vi "HowManyHours.vi"(1 "Error In":errorcluster, 2 "Money":dbl=30.8 format="%#_13g") -> (0 "Info":string)   [LabVIEW 2023]
panel:
  in  "zakończ":bool
  out "Error Out":errorcluster
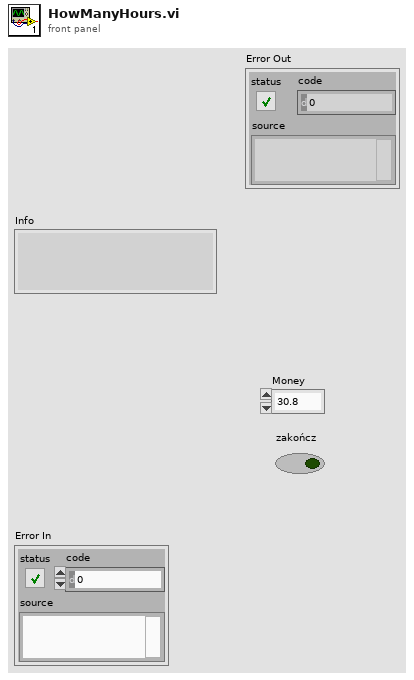
[diagram p1: front panel]
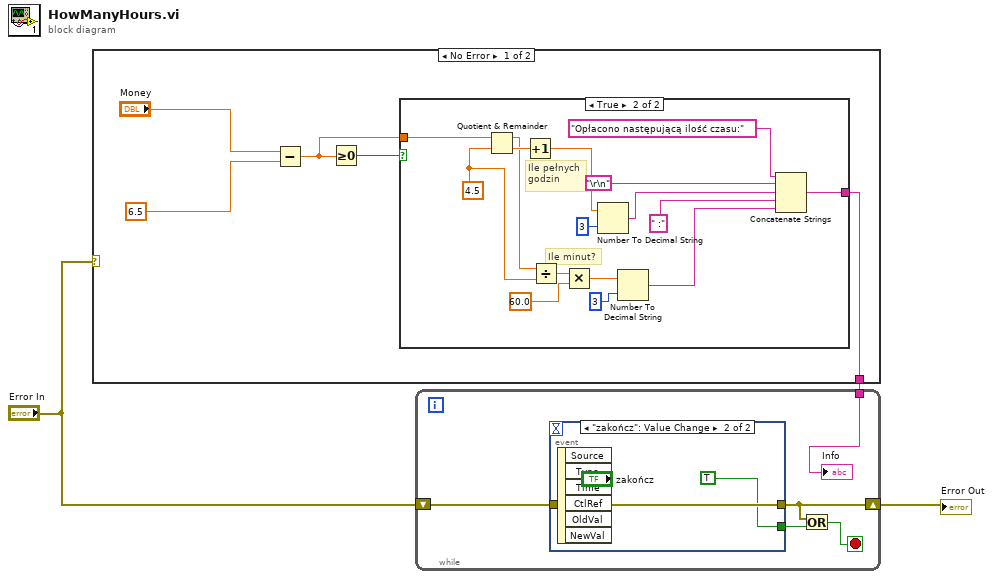
[diagram p0: block diagram]
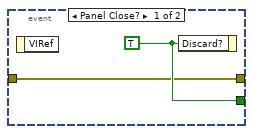
[diagram p2: hidden frame]
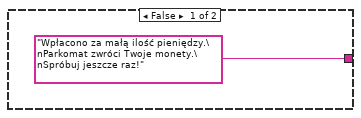
[diagram p3: hidden frame]
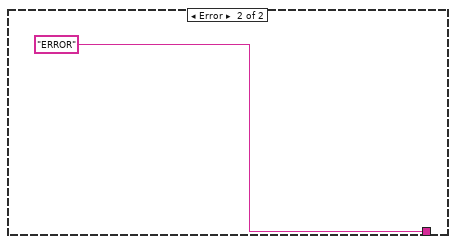
[diagram p4: hidden frame]
diagram:
  n1 = case shown="No Error" "Error In" {
    tunnel: [w4 "ERROR"] -> w3
    frame No Error {
      n2 = Subtract(x="Money", y=6.5) -> (x-y=w5:dbl)
      n3 = Greater Or Equal To 0?(x=w5) -> (x >= 0?=w6:bool)
      n4 = case shown="True" w6 {
        tunnel: w5 -> [_ w25]
        tunnel: ["Wpłacono za małą ilość pieniędzy.\nParkomat zwróci Twoje monety.\nSpróbuj jeszcze raz!" w10] -> w4
        frame False {
        }
        frame True {
          w17 = 4.5 ("y")
          # "Ile pełnych\ngodzin"
          # "Ile minut?"
          n5 = Quotient & Remainder(x=w25, y=w17) -> (x-y*floor(x/y)=w18:dbl, floor(x/y)=w24:dbl)
          n6 = Increment(x=w24) -> (x+1=w20:dbl)
          n7 = Divide(x=w18, y=w17) -> (x/y=w16:dbl)
          n8 = Multiply(x=w16, y=60.0) -> (x*y=w14:dbl)
          n9 = Number To Decimal String(number=w20, width (-)=i16 3) -> (decimal integer string=w23:string)
          n10 = Number To Decimal String(number=w14, width (-)=i16 3) -> (decimal integer string=w12:string)
          n11 = Concatenate Strings("Opłacono następującą ilość czasu:", "\r\n", w23, " :" ("string"), w12) -> (w10:string)
        }
      }
    }
    frame Error {
    }
  }
  n12 = while {
    shift-right: [w27] -> w1
    shift-left: "Error In" -> [w31]
    tunnel: w3 -> [w28]
    stop <- w30 stop-if-true
    n13 = event shown="[1] \"zakończ\": Value Change" {
      selector: _ -> [_ _]
      dyn-events: _ -> [_ _]
      timeout: _ -> [_ _]
      tunnel: w31 -> [w32 w35]
      tunnel: [w32 w35] -> w27
      tunnel: [w33 TRUE ("Discard?")] -> w29
      event Panel Close? {
        w33 = TRUE ("Discard?")
        n14 = event-data() -> ()  [unwired: 1 in, 1 out]
        n15 = event-data("Discard?"=w33) -> ()  [unwired: 1 in, 1 out]
      }
      event "zakończ": Value Change {
        n16 = event-data() -> ()  [unwired: 1 in, 6 out]
      }
    }
    n17 = Or(x=w27, y=w29) -> (x .or. y?=w30:bool)
    "Info" <- w28
  }
  "Error Out" <- w1
